vi "Teardown Created Queues.vi"(11 "Base Queue jettl in":refnum<class "Base Queue jettl.lvclass">) -> (3 "Base Queue jettl out":refnum<class "Base Queue jettl.lvclass">)   [LabVIEW 2021, in "jettl.lvlib" / "Base Queue jettl.lvlib" / "Base Queue jettl.lvclass"]
uses:
  Base Queue jettl.lvclass
  jettl Msg Teardown/Teardown Msg Strategy/Teardown Msg Strategy.lvclass
  C:/git/jettl/src/jettl/Msg Strategy/Msg Strategy.lvclass
  Base Queue jettl.lvclass/Base Queue jettl.ctl
  jettl Msg Teardown/jettl Msg Teardown.lvlib
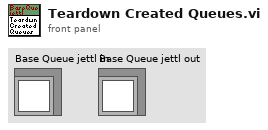
[diagram p1: front panel]
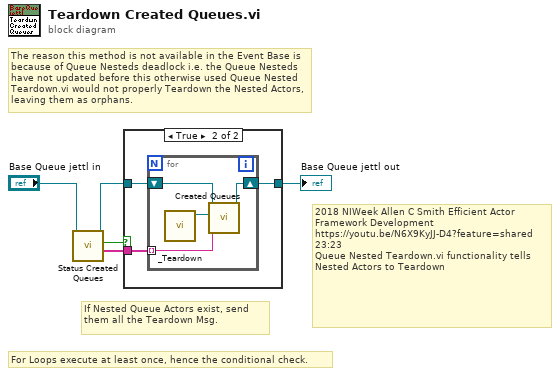
[diagram p0: block diagram]
diagram:
  # "2018 NIWeek Allen C Smith Efficient Actor Framework Development\nhttps://youtu.be/N6X9KyJJ-D4?feature=shared\n23:23\nQueue Nested Teardown.vi functionality tells Nested Actors to Teardown"
  # "For Loops execute at least once, hence the conditional check."
  # "If Nested Queue Actors exist, send them all the Teardown Msg."
  # "The reason this method is not available in the Event Base is because of Queue Nesteds deadlock i.e. the Queue Nesteds have not updated before this otherwise used Queue Nested Teardown.vi would not properly Teardown the Nested Actors, leaving them as orphans."
  n1 = call-dynamic "Status Created Queues.vi"("Base Queue jettl in"="Base Queue jettl in") -> ("Created Queue Aliases"=w1:string[], "Created Queue Exist?"=w2:bool, "Base Queue jettl out"=w3:refnum<class "Base Queue jettl.lvclass">)  [unwired: 7 in, 1 out]
  n2 = case shown="True" w2 {
    tunnel: [w6 w9] -> w5
    tunnel: w3 -> [w6 w8]
    tunnel: w1 -> [_ w7]
    frame False {
    }
    frame True {
      n3 = for {
        tunnel: w7 -> [w12] mode=indexing
        shift-right: [w10] -> w9
        shift-left: w8 -> [w11]
        n4 = call "_Teardown.vi"() -> ("Teardown Msg Strategy out"=w13:refnum<class "Teardown Msg Strategy.lvclass">)  [unwired: 11 in]
        n5 = call-dynamic "Created Queues.vi"("Created Queue Alias"=w12, "Msg Strategy"=w13, "Base Queue jettl in"=w11) -> ("Base Queue jettl out"=w10:refnum<class "Base Queue jettl.lvclass">)  [unwired: 8 in]
      }
    }
  }
  "Base Queue jettl out" <- w5
